vi "ALARMAARDUINO.vi"() -> ()   [LabVIEW 2011]
uses:
  <vilib>/MakerHub/LINX/Public/Peripherals/Digital/Digital Write 1 Chan.vi
  <vilib>/MakerHub/LINX/Public/Peripherals/Digital/Digital Write N Chans.vi
  <vilib>/MakerHub/LINX/Private/Local IO/LinxDigitalWrite.vi
  <vilib>/MakerHub/LINX/Public/Utilities/Check Channel.vi
  <vilib>/MakerHub/LINX/Public/Utilities/Open Serial.vi
  <vilib>/MakerHub/LINX/Private/Utilties/Generate Error.vi
  <vilib>/MakerHub/LINX/LMH-LINX.lvlib
panel:
  in  "DO Channel":u8
  in  "?":bool
  in  "PUERTO SERIAL":refnum<visa-resource-name>="N/A"
  out "VELOCIDAD":u32
  in  "DIA":T1
  out "CONTROL":bool
  out "TIME":timestamp format="%<%H:%M:%S\n%d/%m/%Y>T"
  in  "HORARIO":cluster{"ENCENDIDO":dbl, "APAGADO":dbl} {"APAGADO" format="%<%H:%M>T"; "ENCENDIDO" format="%<%H:%M>T"}
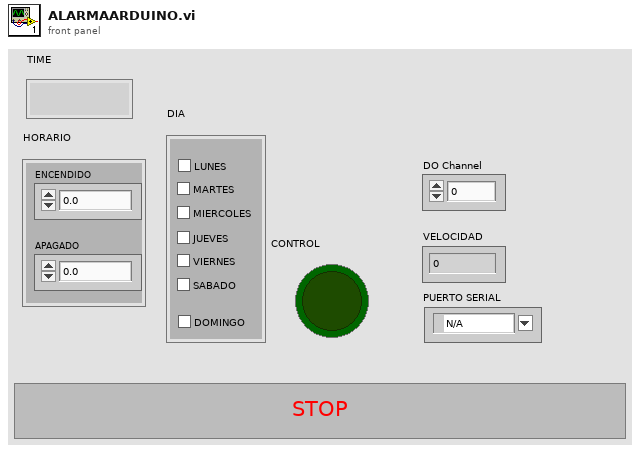
[diagram p1: front panel]
types:
  T1 = cluster{"Boolean":bool, "Boolean 2":bool, "Boolean 3":bool, "Boolean 4":bool, "Boolean 5":bool, "Boolean 6":bool, "Boolean 7":bool}
  T2 = typedef "LMH-LINX.lvlib/LINX Ref.ctl" = cluster{"IO":T3, "Interface":T4, "LINX Device Config":T5}
  T3 = typedef "LMH-LINX.lvlib/Platform.ctl" = enum16{"Remote", "Local"}
  T4 = typedef "LMH-LINX.lvlib/Interface.ctl" = enum16{"Serial", "TCP"}
  T5 = typedef "LMH-LINX.lvlib/Device.lvlib/LINX Device Config.ctl" = cluster{"Interface":T4, "COM Port":refnum<visa-resource-name>, "TCP Configuration":T6, "Device Family":u8, "Device ID":u8, "Device Name":string, "TCP Ref":refnum<k5>, "Channels":T7}
  T6 = typedef "LMH-LINX.lvlib/Device.lvlib/TCP Config.ctl" = cluster{"IP Address":string, "Port":u16}
  T7 = typedef "LMH-LINX.lvlib/Channels.ctl" = cluster{"DI":u8[], "DO":u8[], "AI":u8[], "AO":u8[], "PWM":u8[], "QE":u8[], "UART":u8[], "I2C 2":u8[], "SPI":u8[], "CAN":u8[], "Servo":u8[], "AI Ref (V)":dbl, "AI Resolution (Bits)":u8, "AO Ref (V)":dbl, "AO Resolution (Bits)":u8}
  T8 = typedef "LVDateTimeRec.ctl" = cluster{"fractional second":dbl, "second":i32, "minute":i32, "hour":i32, "day of month":i32, "month":i32, "year":i32, "day of week":i32, "day of year":i32, "DST":i32}
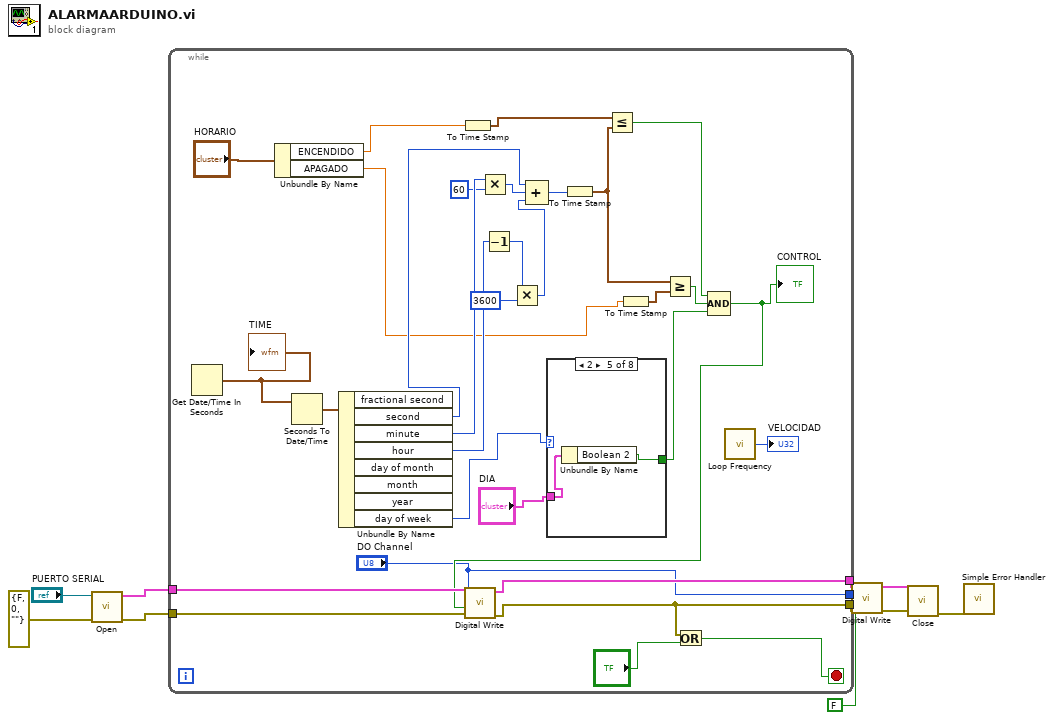
[diagram p0: block diagram]
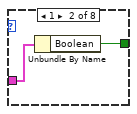
[diagram p3: hidden frame]
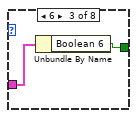
[diagram p4: hidden frame]
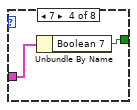
[diagram p5: hidden frame]
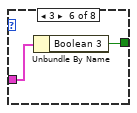
[diagram p6: hidden frame]
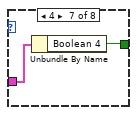
[diagram p7: hidden frame]
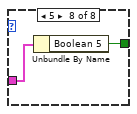
[diagram p8: hidden frame]
diagram:
  n1 = call-poly <vilib>:"Open.vi"("Error In"=errorcluster {"status"=FALSE, "code"=0, "source"=""}, "Serial Port"="PUERTO SERIAL") -> ("Error Out"=w7:errorcluster, "LINX Resource"=w8:T2)  [unwired: 7 in, 1 out]
  n2 = while {
    tunnel: w8 -> [w19]
    tunnel: w7 -> [w18]
    tunnel: [w17] -> w4
    tunnel: [w16] -> w3
    tunnel: ["DO Channel"] -> w1
    stop <- w14 stop-if-true
    n3 = Get Date/Time In Seconds() -> (seconds since 1Jan1904=w41:timestamp)
    "TIME" <- w41
    n4 = Unbundle By Name("HORARIO") -> ("ENCENDIDO"=w29:dbl, "APAGADO"=w28:dbl)
    n5 = Seconds To Date/Time(time stamp (now)=w41) -> (date time rec=w40:T8)  [unwired: 1 in]
    n6 = Unbundle By Name(w40) -> ("second"=w38:i32, "minute"=w37:i32, "hour"=w35:i32, "day of week"=w30:i32)  [unwired: 4 out]
    n7 = To Time Stamp(1:w29) -> (0:w27:timestamp)
    n8 = Multiply(x=w37, y=60) -> (x*y=w32:i32)
    n9 = Decrement(x=w35) -> (x-1=w34:i32)
    n10 = Multiply(x=w34, y=3600) -> (x*y=w31:i32)
    n11 = Compound Arithmetic op=ADD(w38, w32, w31) -> (w39:i32)
    n12 = case shown="2" w30 {
      tunnel: "DIA" -> [_ w44 w45 w48 w49 w51 w53 w55]
      tunnel: [_ w43 w46 w47 w50 w52 w54 w56] -> w21
      frame 0, Default {
      }
      frame 1 {
        n13 = Unbundle By Name(w44) -> ("Boolean"=w43:bool)
      }
      frame 6 {
        n14 = Unbundle By Name(w45) -> ("Boolean 6"=w46:bool)
      }
      frame 7 {
        n15 = Unbundle By Name(w48) -> ("Boolean 7"=w47:bool)
      }
      frame 2 {
        n16 = Unbundle By Name(w49) -> ("Boolean 2"=w50:bool)
      }
      frame 3 {
        n17 = Unbundle By Name(w51) -> ("Boolean 3"=w52:bool)
      }
      frame 4 {
        n18 = Unbundle By Name(w53) -> ("Boolean 4"=w54:bool)
      }
      frame 5 {
        n19 = Unbundle By Name(w55) -> ("Boolean 5"=w56:bool)
      }
    }
    n20 = To Time Stamp(1:w39) -> (0:w25:timestamp)
    n21 = Less Or Equal?(x=w27, y=w25) -> (x <= y?=w24:bool)
    n22 = To Time Stamp(1:w28) -> (0:w26:timestamp)
    n23 = Greater Or Equal?(x=w25, y=w26) -> (x >= y?=w23:bool)
    n24 = Compound Arithmetic op=AND(w24, w23, w21) -> (w13:bool)
    "CONTROL" <- w13
    n25 = call-poly <vilib>:"Digital Write.vi"("Error In"=w18, "Output Value"=w13, "DO Channel"="DO Channel", "LINX Resource"=w19) -> ("Error Out"=w16:errorcluster, "LINX Resource"=w17:T2)  [unwired: 6 in]
    n26 = Or(x=w16, y="?") -> (x .or. y?=w14:bool)
    n27 = call <vilib>:"Loop Frequency.vi"() -> ("Loop Rate (Hz)"=→"VELOCIDAD":u32)
  }
  n28 = call-poly <vilib>:"Digital Write.vi"("Error In"=w3, "Output Value"=FALSE, "DO Channel"=w1, "LINX Resource"=w4) -> ("Error Out"=w11:errorcluster, "LINX Resource"=w10:T2)  [unwired: 6 in]
  n29 = call <vilib>:"Close.vi"("Error In"=w11, "LINX Resource"=w10) -> ("Error Out"=w9:errorcluster)  [unwired: 9 in]
  n30 = call <vilib>:"Simple Error Handler.vi"("error in (no error)"=w9) -> ()  [unwired: 4 in, 5 out]
